vi "State Data.vi"(7 "State":T1) -> (8 "Data":string)   [LabVIEW 2016, in "Centauro.lvlib"]
uses:
  Projects/Centauro.lvlib
  type defs/Machine State.ctl
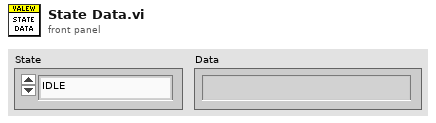
[diagram p1: front panel]
types:
  T1 = typedef "Centauro.lvlib/Machine State.ctl" = enum16{"IDLE", "STANDBY", "DELAY", "RUN", "PAUSE", "DELAY PAUSE", "EOC"}
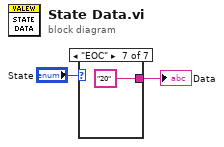
[diagram p0: block diagram]
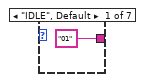
[diagram p2: hidden frame]
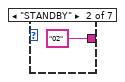
[diagram p3: hidden frame]
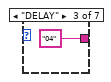
[diagram p4: hidden frame]
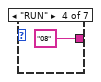
[diagram p5: hidden frame]
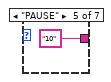
[diagram p6: hidden frame]
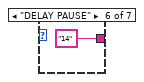
[diagram p7: hidden frame]
diagram:
  n1 = case shown="\"EOC\"" "State" {
    tunnel: ["01" "02" "04" "08" "10" "14" "20"] -> w1
    frame "IDLE", Default {
    }
    frame "STANDBY" {
    }
    frame "DELAY" {
    }
    frame "RUN" {
    }
    frame "PAUSE" {
    }
    frame "DELAY PAUSE" {
    }
    frame "EOC" {
    }
  }
  "Data" <- w1
